vi "Set Menu Button Position.vi"(8 "error in (no error)":errorcluster, 10 "Top Position":i32, 11 "MenuButton in":refnum<class "MenuButton.lvclass">) -> (0 "error out":errorcluster, 2 "Bottom Postion":u32, 3 "MenuButton out":refnum<class "MenuButton.lvclass">)   [LabVIEW 2017, in "MenuButtons.lvlib" / "MenuButton.lvclass"]
uses:
  MenuButton.lvclass
  MenuButton.lvclass/MenuButton.ctl
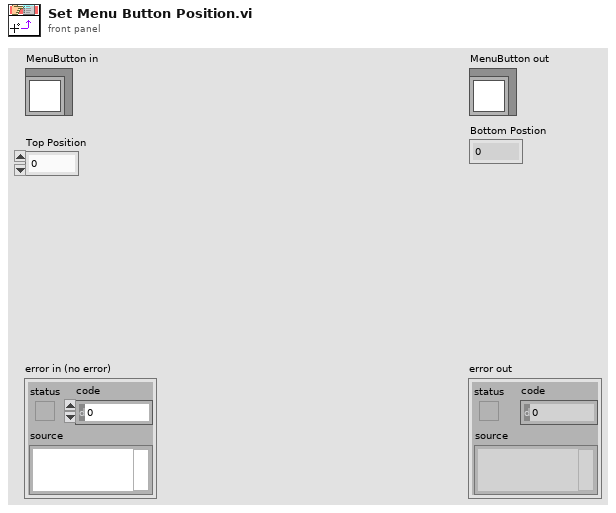
[diagram p1: front panel]
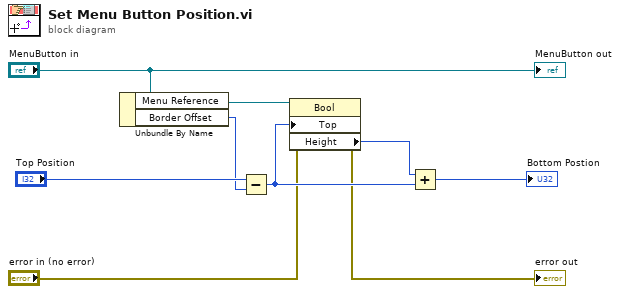
[diagram p0: block diagram]
diagram:
  n1 = Unbundle By Name("MenuButton in") -> ("Menu Reference"=w8:refnum<vi>, "Border Offset"=w6:i32)
  n2 = Subtract(x="Top Position", y=w6) -> (x-y=w5:i32)
  n3 = property class="Bool"(reference=w8, error in="error in (no error)", "Top"=w5) -> (error out=→"error out":errorcluster, "Height"=w4:u32)  [unwired: 1 out]
  n4 = Add(x=w4, y=w5) -> (x+y=→"Bottom Postion":u32)
  "MenuButton out" <- "MenuButton in"
